vi "ap get monitor latency.vi"(9 "dest":cluster{}, 10 "monitor_id":u32, 11 "ap_handle":u32) -> (1 "dest out":cluster{}, 2 "function return":i32, 3 "ap_handle out":u32)   [LabVIEW 2019, in "apdm.lvlib"]
doc: "APDM_EXPORT int apdm_ap_get_monitor_latency(apdm_ap_handle_t ap_handle, const uint32_t monitor_id, int64_t *dest);"
uses:
  apdm.lvlib
  Lee Lab/CP FES Walking 2018/Code/Working/LabVIEW/apdm.dll
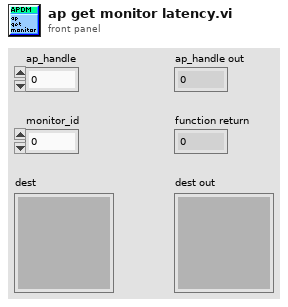
[diagram p1: front panel]
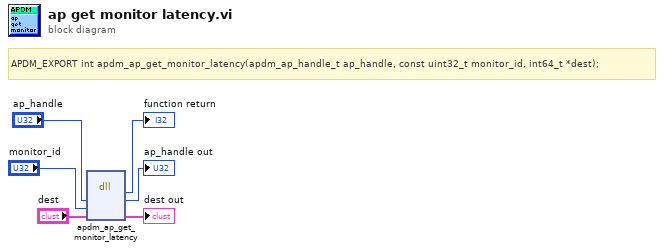
[diagram p0: block diagram]
diagram:
  # "APDM_EXPORT int apdm_ap_get_monitor_latency(apdm_ap_handle_t ap_handle, const uint32_t monitor_id, int64_t *dest);"
  n1 = dll-call lib="C:/Users/jfalesi/Dropbox/Lee Lab/CP FES Walking 2018/Code/Working/LabVIEW/apdm.*" fn="apdm_ap_get_monitor_latency"("ap_handle"="ap_handle", "monitor_id"="monitor_id", "dest"="dest") -> (→"function return":i32, "ap_handle"=→"ap_handle out":u32, "dest"=→"dest out":cluster{})  [unwired: 4 in, 2 out]
